vi "Event handler-Load ref image.vi"() -> (0 "error out":errorcluster, 3 "Error or cancelled":bool)   [LabVIEW 2020]
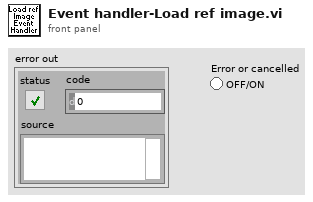
[diagram p1: front panel]
types:
  T1 = typedef "Imaging Protocols enum.ctl" = enum16{"AOL Z-Stack", "Motor Z Stack", "Functional Acquisition", "Single Plane Acquisition", "Volume Acquisition", "Live Imaging", "Live Plane Imaging", "Live Volume Imaging"}
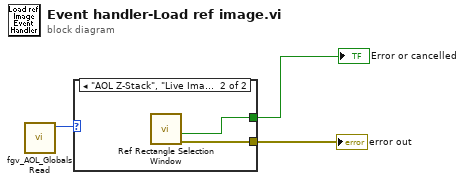
[diagram p0: block diagram]
diagram:
  n1 = call "fgv_AOL_Globals Read.vi"() -> ("Imaging Protocol"=w3:T1)  [unwired: 9 in, 2 out]
  n2 = case shown="\"AOL Z-Stack\", \"Live Imaging\"" w3 {
    tunnel: [_ w5] -> w1
    tunnel: [_ w4] -> w2
    frame Default {
    }
    frame "AOL Z-Stack", "Live Imaging" {
      n3 = call "Ref Rectangle Selection Window.vi"() -> ("error out"=w5:errorcluster, "Error or cancelled"=w4:bool)  [unwired: 10 in]
    }
  }
  "error out" <- w1
  "Error or cancelled" <- w2
